vi "What Is Love (LV2013).vi"   [LabVIEW 2013]
uses:
  <vilib>/sound2/lvsound2.llb/Sampling Mode.ctl
  <vilib>/sound2/lvsound2.llb/Sound Output Write (I16).vi
types:
  T1 = typedef "Sampling Mode.ctl" = i32
  T2 = cluster{"sample rate (S/s)":dbl, "number of channels":i32, "bits per sample":i32}
  T3 = typedef "Sound Output Task ID.ctl" = u32
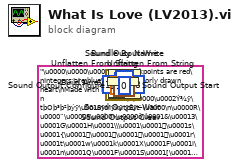
[diagram p0: block diagram]
diagram:
  n1 = Unflatten From String(type=u8[] [], binary string="\u0000\u0000\u0000  \nBreakpoints are red\nIntegers are blue\nHere's a poorly drawn heart\nMade with LabVIEW\n                                         \n\u0000\u0002Ý¾ÿ\tþOþ³þ²þýÿ\u0015ÿMÿkÿ ÿÊÿ÷\u0000\n\u0000R\u0000¨\u0000¶\u0000»\u0000ô\u0001&\u00013\u0001G\u0001H\u0001\\\u0001\u0001\u0001s\u0001{\u0001\u0001\u0001\u0001\u0001r\u0001t\u0001w\u0001k\u0001X\u0001F\u0001i\u0001n\u0001Q\u0001F\u0001S\u0001[\u0001g\u0001V\u0001T\u0001e\u0001l\u0001W\u00019\u0001'\u0001-\u0001\r\u0001\u000b\u0001\u0004\u0000â\u0000Ù\u0000¯\u0000\u0000y\u0000\\\u00009\u0000\u0012ÿýÿÑÿÿÿlÿQÿ*ÿ\u0005þçþÎþ®þ~þjþmþsþjþcþZþþþ þ¦þ¥þÂþÓþàþíþóþðÿ\u0000þñþðÿ\bþôþïÿ\u0013ÿ\u000eÿ\u0011ÿ\nþýÿ\u0017ÿ'ÿ%ÿ\u0017ÿ\u0018ÿ\"ÿ\u001aÿ\u0019þäþáÿ\fþ÷þôþÜþãþüþÿþ÷ÿ\u000eÿEÿ`ÿ<ÿ2ÿÿÄÿ¾ÿÍÿÖ\u0000\u0003\u0000#\u0000\u000b\u0000\nÿúÿßÿ®ÿ`ÿDÿ&þÍþþ\u0019ýÀýýwýNý\u0012ý3ýSý`ýXýFýkýý¨ý¼ýéþ\u0007þ*þ.þPþþÄþòÿ\u0014ÿ@ÿuÿÿÆ\u0000\u0002\u0000=\u0000[\u0000x\u0000£\u0000Í\u0000â\u0000Ó\u0000ç\u0001\u000f\u0001D\u0001J\u0001;\u0001B\u0001\\\u0001i\u0001c\u0001e\u0001\\\u0001g\u0001n\u0001w\u0001g\u0001q\u0001\u0001\u0001s\u0001s\u0001n\u0001\u0001\u0001~\u0001£\u0001ª\u0001¥\u0001¡\u0001°\u0001©\u0001¨\u0001\u0001\u0001\u0001\u0001z\u0001p\u0001i\u00019\u0001\u0014\u0000ö\u0000Ú\u0000¸\u0000\u0000M\u00009\u0000\u001bÿèÿ¬ÿÿ]ÿQÿIÿ..." ("concatenated string")) -> (rest of the binary string=w8:string)  [unwired: 3 in, 2 out]
  n2 = call <vilib>:"Sound Output Configure.vi"("number of samples/ch"=187838, "sample mode"=T1 0, "sound format"=T2 {"sample rate (S/s)"=22050.0, "number of channels"=1, "bits per sample"=16}) -> ("error out"=w19:errorcluster, "task ID"=w20:T3)  [unwired: 7 in]
  n3 = call <vilib>:"Sound Output Start.vi"("error in (no error)"=w19, "task ID"=w20) -> ("error out"=w18:errorcluster, "task ID out"=w16:T3)  [unwired: 8 in]
  n4 = Unflatten From String(type=i16[] [], binary string=w8, error in (no error)=w18) -> (value=w5:i16[], error out=w17:errorcluster)  [unwired: 2 in, 1 out]
  n5 = Bundle By Name("Y"=w5) -> (w4:waveform(i16))  [unwired: 1 in]
  n6 = Build Array(w4) -> (w3:waveform(i16)[])
  n7 = call-poly <vilib>:"Sound Output Write.vi"("timeout (sec)"=10.0, "error in (no error)"=w17, "data"=w3, "task ID"=w16) -> ("error out"=w12:errorcluster, "task ID out"=w13:T3)  [unwired: 6 in]
  n8 = call <vilib>:"Sound Output Wait.vi"("error in (no error)"=w12, "task ID"=w13) -> ("error out"=w10:errorcluster, "task ID out"=w11:T3)  [unwired: 8 in]
  n9 = call <vilib>:"Sound Output Clear.vi"("error in (no error)"=w10, "task ID"=w11) -> ()  [unwired: 9 in, 1 out]
